vi "Load Certificate File.vi"(8 "error in (no error)":errorcluster, 11 "CIF_UI in":refnum<class "CIF_UI.lvclass">) -> (0 "error out":errorcluster, 3 "CIF_UI out":refnum<class "CIF_UI.lvclass">)   [LabVIEW 2021, in "CIF_UI.lvclass"]
uses:
  CIF_UI.lvclass
  CIF_UI.lvclass/CIF_UI.ctl
  CIFUtilities/CIFConfigurationFile/CIF Configuration File.lvlib
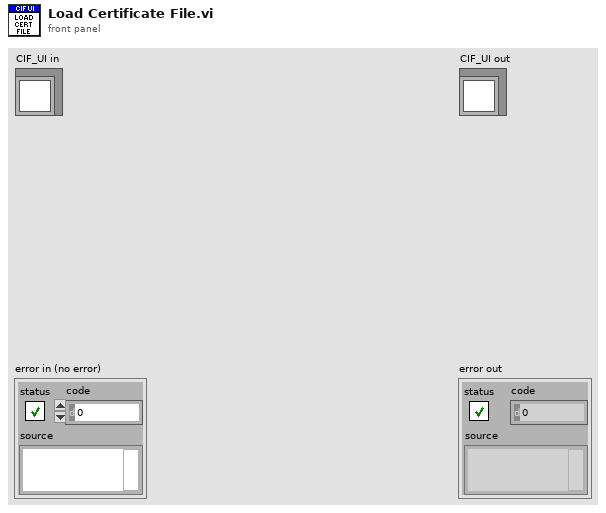
[diagram p1: front panel]
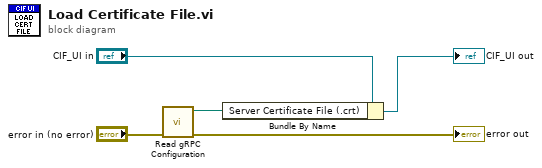
[diagram p0: block diagram]
diagram:
  n1 = call "Read gRPC Configuration.vi"("error in"="error in (no error)") -> ("error out"=→"error out":errorcluster, "Server Certificate File (.crt)"=w1:path)  [unwired: 5 in, 4 out]
  n2 = Bundle By Name(cluster="CIF_UI in", "Server Certificate File (.crt)"=w1) -> (→"CIF_UI out":refnum<class "CIF_UI.lvclass">)
